vi "Test Warning to Error Handler.vi"() -> ()   [LabVIEW 2013]
uses:
  source/State Machine Support API/Select State(s)_err.vi
  source/State Machine Support API/Select State(s)_bool.vi
  <userlib>/_OpenG.lib/numeric/numeric.llb/Random Number Within Range - I32__ogtk.vi
panel:
  in  "Include Call Chain":bool
  in  "Generate Error":bool
  in  "Generate Warning":bool
  out "Previous Arguments":string
  out "Previous States":string
  out "Error message":string
  in  "Exit":bool
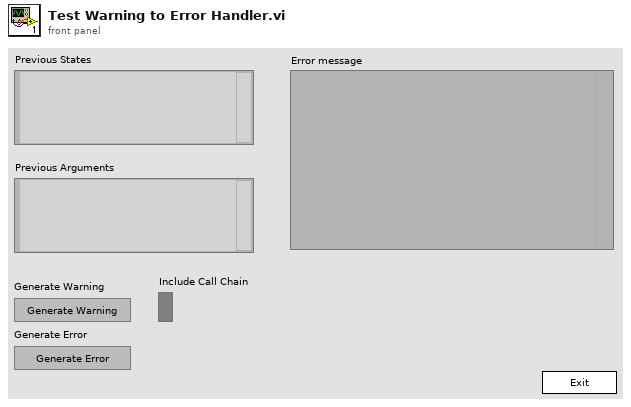
[diagram p1: front panel]
types:
  T1 = enum32{"Invalid", "Standard", "Closed", "Hidden", "Minimized", "Maximized"}
  T2 = enum32{"invalid app kind", "Development System", "Run Time System", "Student Edition", "Embedded LabVIEW", "Evaluation", "Custom"}
  T3 = cluster{"Core":cluster{"Current VI Reference":refnum<vi>, "Close Panel on Exit?":bool}, "Your Boolean data":bool, "Your string data":string}
  T4 = cluster{"Current VI Reference":refnum<vi>, "Close Panel on Exit?":bool}
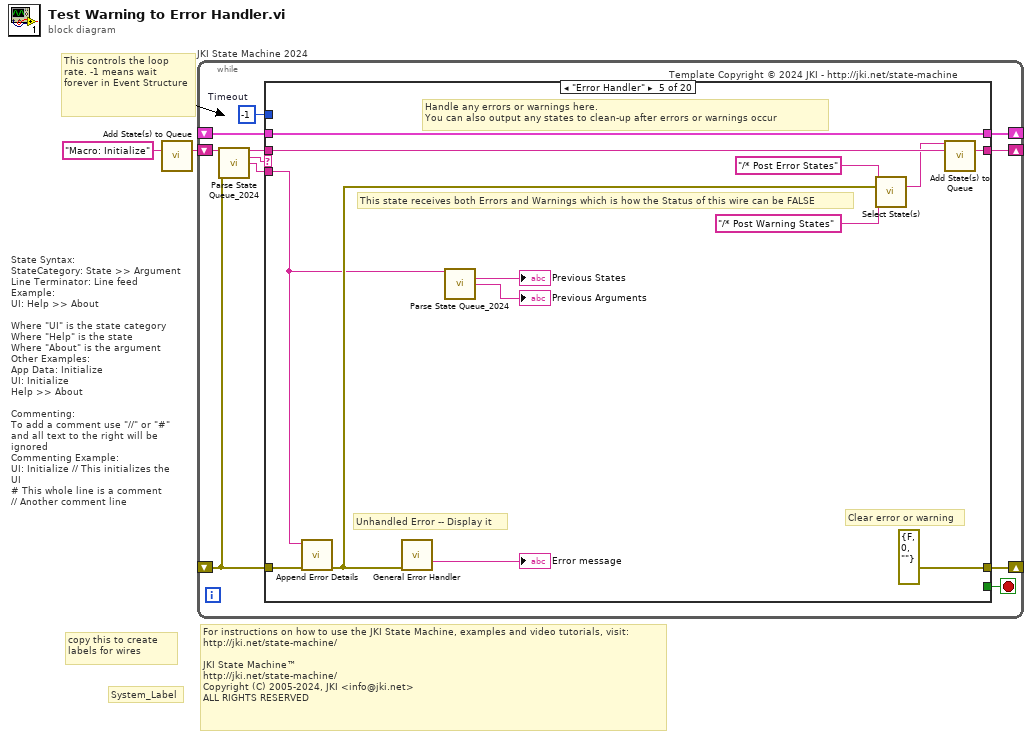
[diagram p0: block diagram]
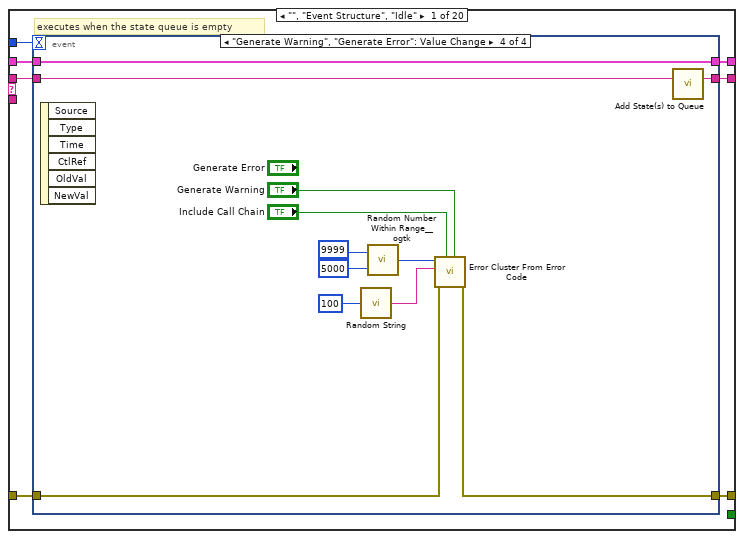
[diagram p2: hidden frame]
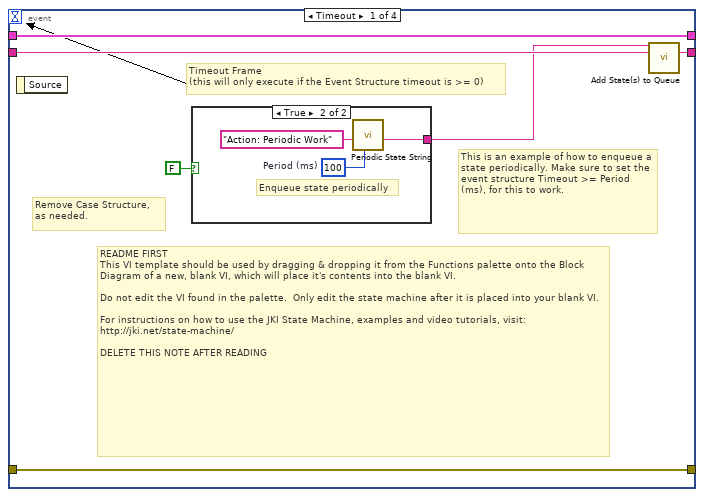
[diagram p3: hidden frame]
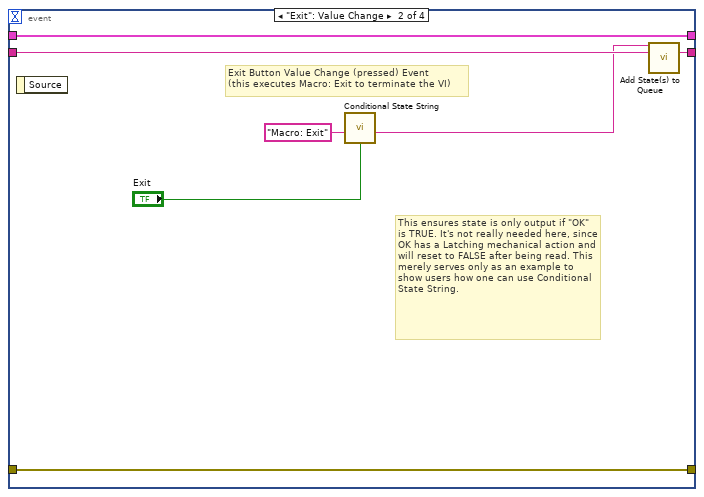
[diagram p5: hidden frame]
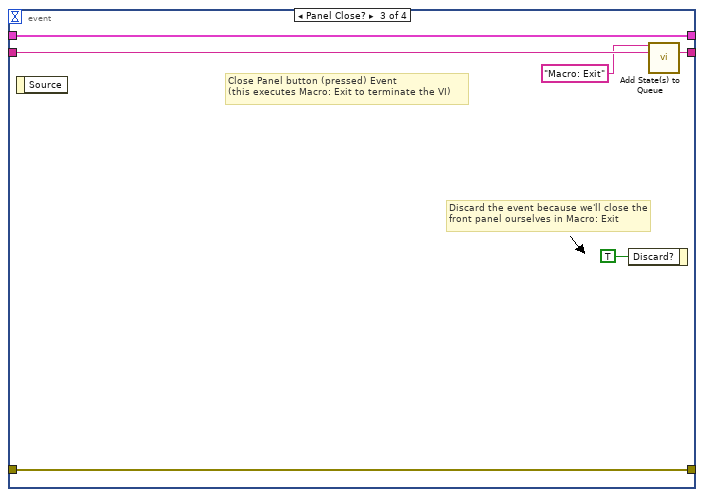
[diagram p6: hidden frame]
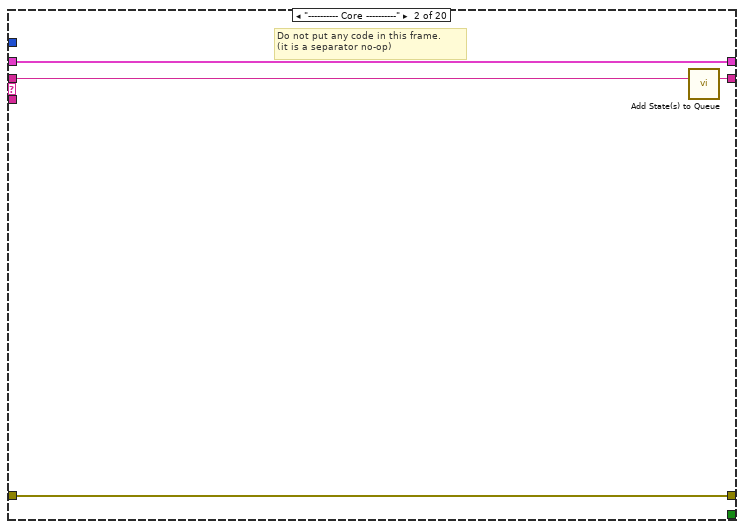
[diagram p7: hidden frame]
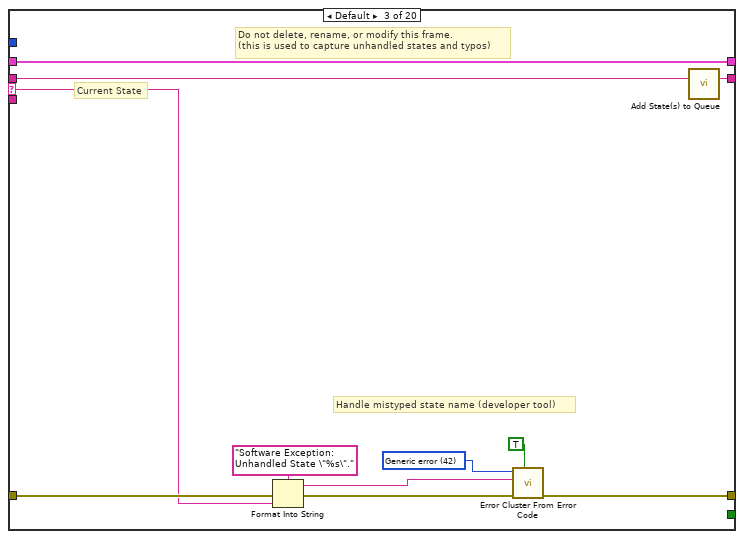
[diagram p8: hidden frame]
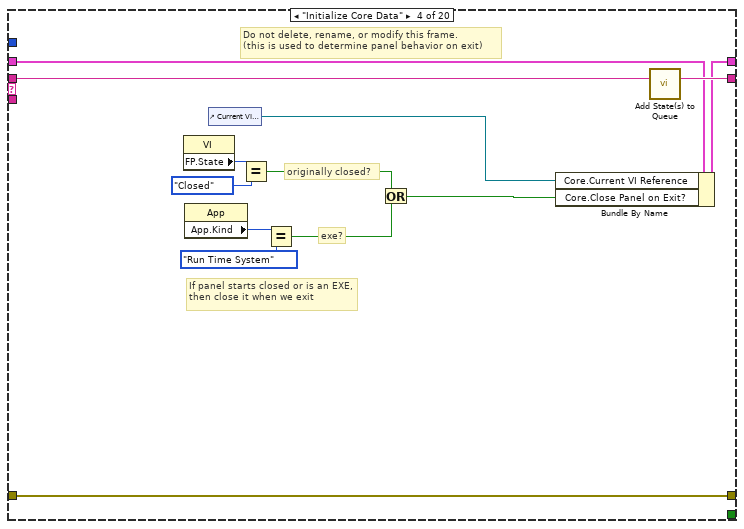
[diagram p9: hidden frame]
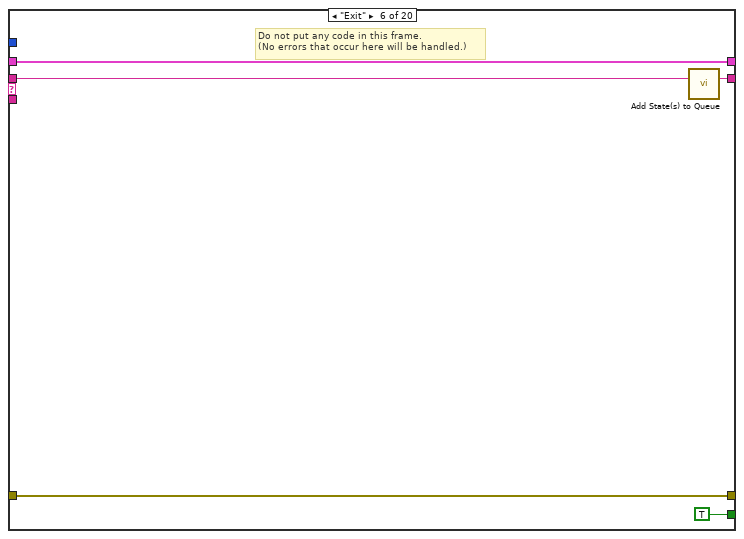
[diagram p10: hidden frame]
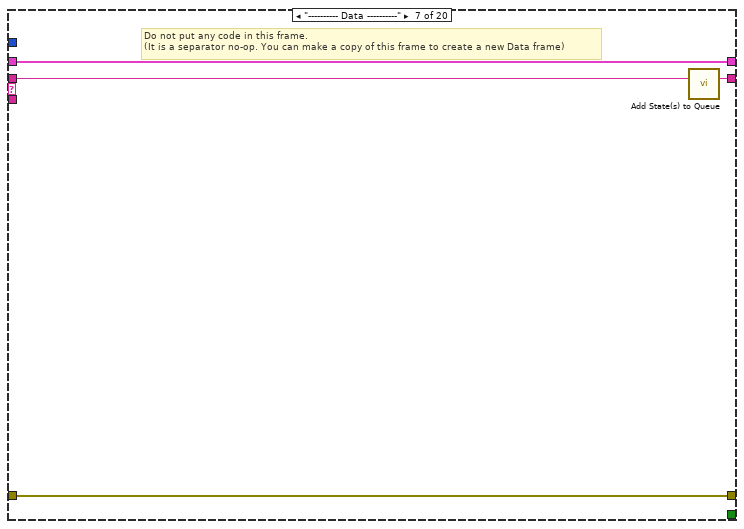
[diagram p11: hidden frame]
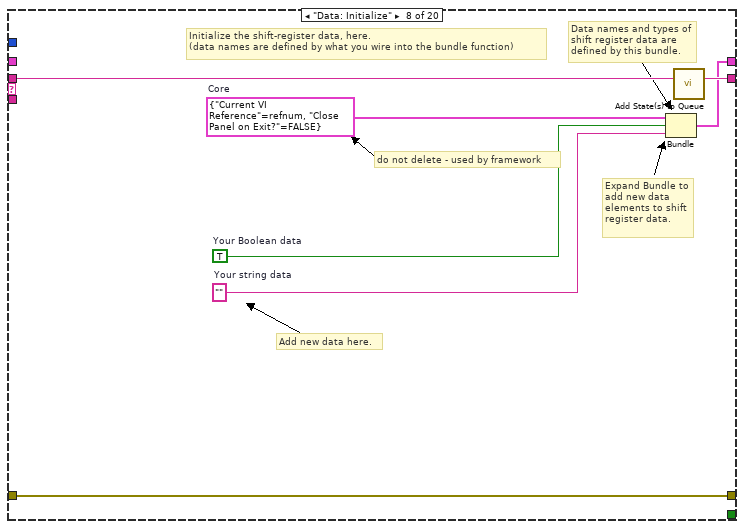
[diagram p12: hidden frame]
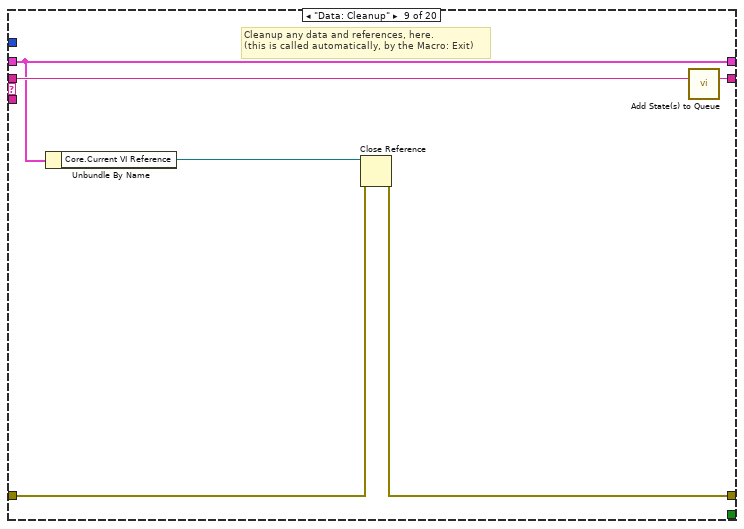
[diagram p13: hidden frame]
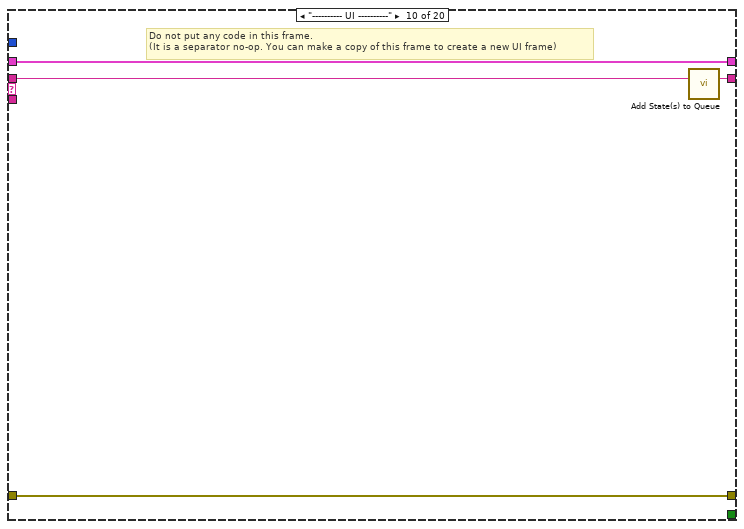
[diagram p14: hidden frame]
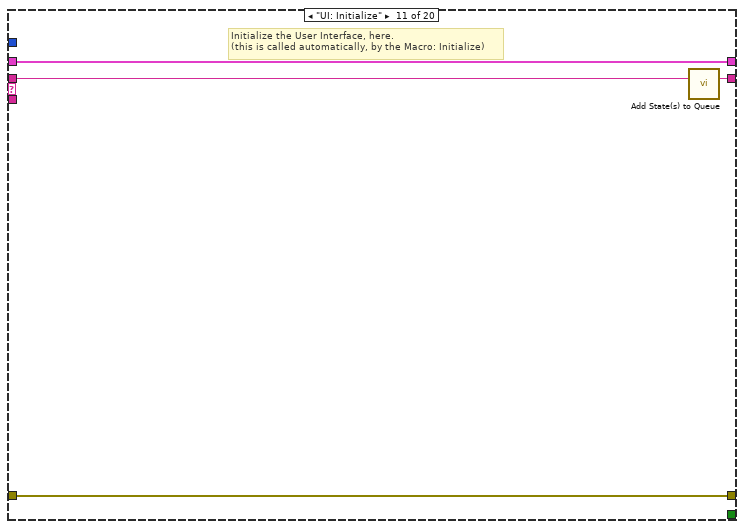
[diagram p15: hidden frame]
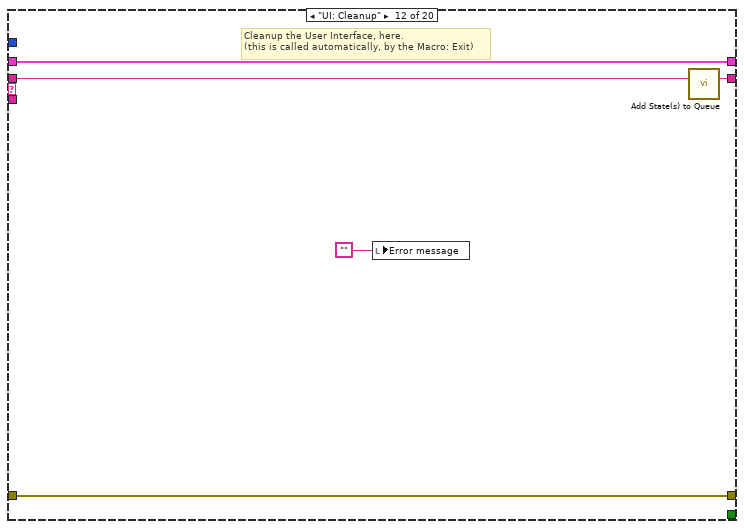
[diagram p16: hidden frame]
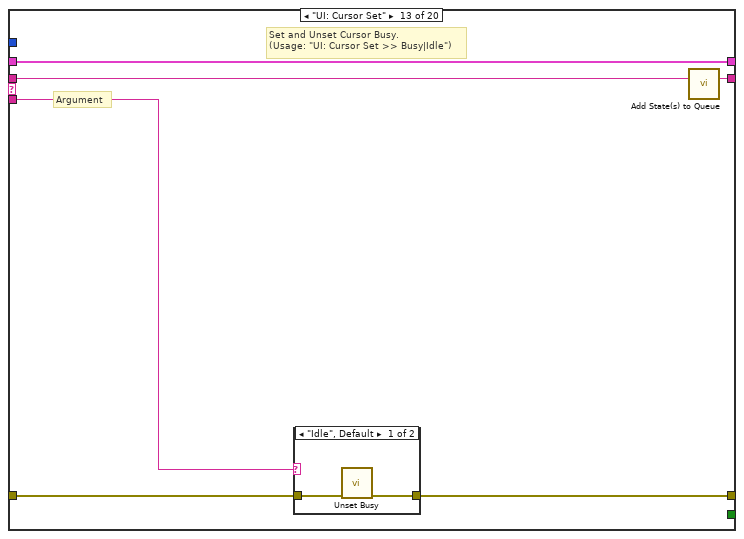
[diagram p17: hidden frame]
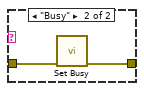
[diagram p18: hidden frame]
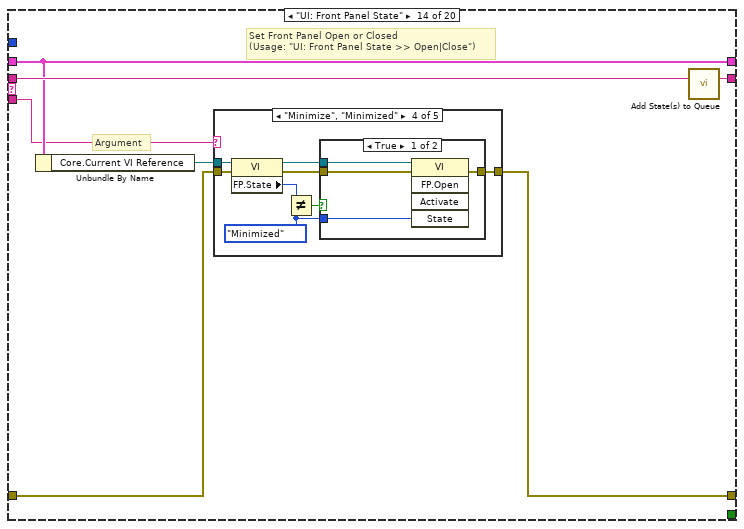
[diagram p19: hidden frame]
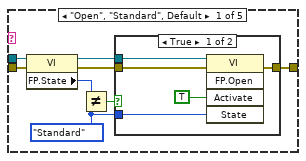
[diagram p20: hidden frame]
diagram:
  # "For instructions on how to use the JKI State Machine, examples and video tutorials, visit:\nhttp://jki.net/state-machine/\n\nJKI State Machine™\nhttp://jki.net/state-machine/\nCopyright (C) 2005-2024, JKI <info@jki.net>\nALL RIGHTS RESERVED"
  # "State Syntax:\nStateCategory: State >> Argument\nLine Terminator: Line feed\nExample:\nUI: Help >> About\n\nWhere \"UI\" is the state category\nWhere \"Help\" is the state\nWhere \"About\" is the argument\nOther Examples:\nApp Data: Initialize\nUI: Initialize\nHelp >> About\n\nCommenting:\nTo add a comment use \"//\" or \"#\" and all text to the right will be ignored\nCommenting Example:\nUI: Initialize // This initializes the UI\n# This whole line is a comment\n// Another comment line"
  # "copy this to create labels for wires"
  # "This controls the loop rate. -1 means wait forever in Event Structure"
  # "System_Label"
  n1 = call "Add State(s) to Queue.vi"("State(s) in (\"\")"="Macro: Initialize") -> ("States Out"=w1:string)  [unwired: 14 in]
  n2 = while "JKI State Machine 2024" {
    shift-right: [w6] -> _
    shift-left: _ -> [w5]
    shift-right: [w9] -> _
    shift-left: _ -> [w3]
    shift-right: [w8] -> _
    shift-left: w1 -> [w10]
    stop <- w7 stop-if-true
    w4 = -1  # Timeout
    # "Template Copyright © 2024 JKI - http://jki.net/state-machine"
    n3 = call "Parse State Queue_2024.vi"("State Queue"=w10, "Error In (no error)"=w3) -> ("Remaining States"=w12:string, "Current State"=w13:string, "Arguments"=w11:string)  [unwired: 11 in]
    n4 = case shown="\"Error Handler\"" w13 {
      selector: w13 -> [_ _ w59 _ _ _ _ _ _ _ _ _ _ _ _ _ _ _ _ _]
      tunnel: w12 -> [w20 w58 w63 w82 w95 w100 w104 w111 w117 w121 w125 w130 w136 w147 w216 w221 w230 w234 w238 w242]
      tunnel: w11 -> [_ _ _ _ w85 _ _ _ _ _ _ _ w131 w141 _ _ _ _ _ _]
      tunnel: w5 -> [w18 w55 w61 w75 w92 w98 w101 _ w112 w118 w123 w128 w134 w143 w213 w218 w228 w231 w235 w239]
      tunnel: [w17 w56 w65 w79 errorcluster {"status"=FALSE, "code"=0, "source"=""} ("error out") w97 w102 w108 w113 w119 w122 w127 w132 w144 w214 w219 w225 w232 w236 w240] -> w9
      tunnel: w3 -> [w14 w56 w64 w79 w91 w97 w102 w108 w114 w119 w122 w127 w133 w145 w214 w219 w225 w232 w236 w240]
      tunnel: [w19 w57 w62 w81 w94 w99 w103 w110 w116 w120 w124 w129 w135 w146 w215 w220 w229 w233 w237 w241] -> w8
      tunnel: [_ _ _ _ _ TRUE _ _ _ _ _ _ _ _ _ _ _ _ _ _] -> w7
      tunnel: [w16 w55 w61 w80 w92 w98 w101 w109 w112 w118 w123 w128 w134 w143 w213 w218 w228 w231 w235 w239] -> w6
      tunnel: w4 -> [w15 _ _ _ _ _ _ _ _ _ _ _ _ _ _ _ _ _ _ _]
      frame "", "Event Structure", "Idle" {
        # "executes when the state queue is empty"
        n5 = event shown="[3] \"Generate Warning\", \"Generate Error\": Value Change" {
          selector: _ -> [_ _ _ _]
          dyn-events: _ -> [_ _ _ _]
          timeout: w15 -> [_ _ _ _]
          tunnel: w20 -> [w26 w36 w42 w54]
          tunnel: [w25 w35 w41 w53] -> w19
          tunnel: w18 -> [w23 w33 w39 w52]
          tunnel: [w24 w34 w40 w48] -> w17
          tunnel: w14 -> [w24 w34 w40 w49]
          tunnel: [w23 w33 w39 w52] -> w16
          event Timeout {
            # "Remove Case Structure, as needed."
            # "This is an example of how to enqueue a state periodically. Make sure to set the event structure Timeout >= Period (ms), for this to work."
            # "README FIRST\nThis VI template should be used by dragging & dropping it from the Functions palette onto the Block Diagram of a new, blank VI, which will place it's contents into the blank VI.\n\nDo not edit the VI found in the palette.  Only edit the state machine after it is placed into your blank VI.\n\nFor instructions on how to use the JKI State Machine, examples and video tutorials, visit:\nhttp://jki.net/state-machine/\n\nDELETE THIS NOTE AFTER READING"
            # "Timeout Frame\n(this will only execute if the Event Structure timeout is >= 0)"
            n6 = event-data() -> ()  [unwired: 1 in, 1 out]
            n7 = case shown="True" FALSE {
              tunnel: [_ w29] -> w22
              frame False {
              }
              frame True {
                w27 = u32 100  # Period (ms)
                # "Enqueue state periodically"
                n8 = call "Periodic State String.vi"("Period (ms)"=w27, "State"="Action: Periodic Work") -> ("State Out"=w29:string)  [unwired: 9 in]
              }
            }
            n9 = call "Add State(s) to Queue.vi"("State(s) in Front (\"\")"=w22, "State(s) in (\"\")"=w26) -> ("States Out"=w25:string)  [unwired: 13 in]
          }
          event "Exit": Value Change {
            # "This ensures state is only output if \"OK\" is TRUE. It's not really needed here, since OK has a Latching mechanical action and will reset to FALSE after being read. This merely serves only as an example to show users how one can use Conditional State String."
            # "Exit Button Value Change (pressed) Event\n(this executes Macro: Exit to terminate the VI)"
            n10 = event-data() -> ()  [unwired: 1 in, 1 out]
            n11 = call "Conditional State String.vi"("Do State(s)?"="Exit", "State"="Macro: Exit") -> ("State Out"=w30:string)  [unwired: 7 in]
            n12 = call "Add State(s) to Queue.vi"("State(s) in Front (\"\")"=w30, "State(s) in (\"\")"=w36) -> ("States Out"=w35:string)  [unwired: 13 in]
          }
          event Panel Close? {
            # "Discard the event because we'll close the front panel ourselves in Macro: Exit"
            # "Close Panel button (pressed) Event\n(this executes Macro: Exit to terminate the VI)"
            n13 = event-data() -> ()  [unwired: 1 in, 1 out]
            n14 = event-data("Discard?"=TRUE) -> ()  [unwired: 1 in, 1 out]
            n15 = call "Add State(s) to Queue.vi"("State(s) in Front (\"\")"="Macro: Exit", "State(s) in (\"\")"=w42) -> ("States Out"=w41:string)  [unwired: 13 in]
          }
          event "Generate Warning", "Generate Error": Value Change {
            n16 = event-data() -> ()  [unwired: 1 in, 6 out]
            n17 = call "Random String.vi"("Length"=100) -> ("ASCII"=w44:string)  [unwired: 4 in]
            n18 = call-poly <userlib>:"Random Number Within Range__ogtk.vi"("High"=9999, "Low"=5000) -> ("Random Number"=w45:i32)  [unwired: 3 in]
            n19 = call <vilib>:"Error Cluster From Error Code.vi"("is warning? (False)"="Generate Warning", "show call chain? (False)"="Include Call Chain", "error in (no error)"=w49, "error message (\"\")"=w44, "error code (0)"=w45) -> ("error out"=w48:errorcluster)  [unwired: 4 in]
            n20 = call "Add State(s) to Queue.vi"("State(s) in (\"\")"=w54) -> ("States Out"=w53:string)  [unwired: 14 in]
          }
        }
      }
      frame "---------- Core ----------" {
        # "Do not put any code in this frame.\n(it is a separator no-op)"
        n21 = call "Add State(s) to Queue.vi"("State(s) in (\"\")"=w58) -> ("States Out"=w57:string)  [unwired: 14 in]
      }
      frame Default {
        w68 = 42 items=["No error", "Argument error", "Memory is full", "Out of zone", "End of file", "File already open", "Generic file I/O error", "File not found", "File permission error", "Disk is full", "Duplicate path", "Too many files open", "System feature not enabled", "Resource file not found", "Cannot add resource", "Resource not found", "Image not found", "Image memory error", "Pen does not exist", "Config type invalid", "Config token not found", "Config parse error", "Config memory error", "Bad external code format", "Bad external code offset", "External code not present", "Null window", "Destroy window error", "Null menu", "Print aborted", "Bad print record", "Print driver error", "Windows error during printing", "Memory error during printing", "Print dialog error", "Generic print error", "Invalid device refnum", "Device not found", "Device parameter error", "Device unit error", "Cannot open device", "Device call aborted", "Generic error", "Cancelled by user", "Object ID too low", "Object ID too high", "Object not in heap", "Unknown heap", "Unknown object (invalid DefProc)", "Unknown object (DefProc not in table)", "Message out of range", "Invalid (null) method", "Unknown message", "Manager call not supported", "Bad address", "Network operation in progress", "Network operation timed out", "Connection is busy", "Network attribute not supported", "Network error", "Address in use", "System out of memory", "Connection aborted", "Connection refused", "Not connected", "Already connected", "Connection closed", "Initialization error (interapplication manager)", "Bad occurrence", "Wait on unbound occurrence handler", "Occurrence queue overflow", "Datalog type conflict", "Unused", "Unrecognized type (interapplication manager)", "Memory corrupt", "Failed to make temporary DLL", "Old CIN version", "Drag socket not found", "Failed to load drop-object", "Failed to register OLE object", "Failed to release OLE object", "Format specifier type mismatch", "Unknown format specifier", "Too few format specifiers", "Too many format specifiers", "Scan failed", "Newer CIN version", "Error converting to variant", "Runtime menu error", "Password tampered", "Variant attribute not found", "Incompatible variant data type", "Event data is not available", "Event Store is not present", "Occurrence is not found", "Event Queue is not created", "Event info is not available", "Refnum passed is NULL", "Error retrieving Class GUID", "Error retrieving CoClass GUID", "Error retrieving TypeLib GUID.", "Bad built application magic bytes.", "Specific driver is different from the specific driver associated with the Logical Name.", "There is no session opened to the class driver.", "Max Error", "MAX - Error with config objects", "MAX - Error loading configuration", "MAX - Group not supported"]
        # "Current State"
        # "Do not delete, rename, or modify this frame.\n(this is used to capture unhandled states and typos)"
        # "Handle mistyped state name (developer tool)"
        n22 = Format Into String(format string="Software Exception: Unhandled State \"%s\"." ("message"), error in=w64, w59) -> (resulting string=w67:string, error out=w66:errorcluster)  [unwired: 1 in]
        n23 = call <vilib>:"Error Cluster From Error Code.vi"("show call chain? (False)"=TRUE, "error in (no error)"=w66, "error message (\"\")"=w67, "error code (0)"=w68) -> ("error out"=w65:errorcluster)  [unwired: 5 in]
        n24 = call "Add State(s) to Queue.vi"("State(s) in (\"\")"=w63) -> ("States Out"=w62:string)  [unwired: 14 in]
      }
      frame "Initialize Core Data" {
        # "Do not delete, rename, or modify this frame.\n(this is used to determine panel behavior on exit)"
        # "originally closed?"
        # "exe?"
        # "If panel starts closed or is an EXE, then close it when we exit"
        n25 = property class="VI"() -> ("FP.State"=w72:T1)  [unwired: 2 in, 2 out]
        n26 = property class="App"() -> ("App.Kind"=w78:T2)  [unwired: 2 in, 2 out]
        n27 = control-ref of="Current VI Reference"() -> (w73:refnum<vi>)
        n28 = Equal?(x=w72, y=T1."Closed" ("Front Panel Window:State")) -> (x = y?=w70:bool)
        n29 = Equal?(x=w78, y=T2."Run Time System" ("Application:Kind")) -> (x = y?=w76:bool)
        n30 = Or(x=w70, y=w76) -> (x .or. y?=w74:bool)
        n31 = Bundle By Name(cluster=w75, "Core.Current VI Reference"=w73, "Core.Close Panel on Exit?"=w74) -> (w80:T3)
        n32 = call "Add State(s) to Queue.vi"("State(s) in (\"\")"=w82) -> ("States Out"=w81:string)  [unwired: 14 in]
      }
      frame "Error Handler" {
        # "This state receives both Errors and Warnings which is how the Status of this wire can be FALSE"
        # "Unhandled Error -- Display it"
        # "Handle any errors or warnings here.\nYou can also output any states to clean-up after errors or warnings occur"
        # "Clear error or warning"
        n33 = call "Append Error Details.vi"("error in (no error)"=w91, "Previous State and Argument(s)"=w85) -> ("error out"=w90:errorcluster)  [unwired: 9 in]
        n34 = call <vilib>:"General Error Handler.vi"("error in (no error)"=w90) -> ("message"=→"Error message":string)  [unwired: 10 in, 4 out]
        n35 = call "Parse State Queue_2024.vi"("State Queue"=w85) -> ("Current State"=→"Previous States":string, "Arguments"=→"Previous Arguments":string)  [unwired: 12 in, 1 out]
        n36 = call-poly "Select State(s).vi"("State(s) if True (\"\")"="/* Post Error States", "Select"=w90, "State(s) if False (\"\")"="/* Post Warning States") -> ("States Out"=w88:string)  [unwired: 12 in]
        n37 = call "Add State(s) to Queue.vi"("State(s) in Front (\"\")"=w88, "State(s) in (\"\")"=w95) -> ("States Out"=w94:string)  [unwired: 13 in]
      }
      frame "Exit" {
        # "Do not put any code in this frame.\n(No errors that occur here will be handled.)"
        n38 = call "Add State(s) to Queue.vi"("State(s) in (\"\")"=w100) -> ("States Out"=w99:string)  [unwired: 14 in]
      }
      frame "---------- Data ----------" {
        # "Do not put any code in this frame.\n(It is a separator no-op. You can make a copy of this frame to create a new Data frame)"
        n39 = call "Add State(s) to Queue.vi"("State(s) in (\"\")"=w104) -> ("States Out"=w103:string)  [unwired: 14 in]
      }
      frame "Data: Initialize" {
        w105 = T4 {"Current VI Reference"=refnum, "Close Panel on Exit?"=FALSE}  # Core
        w107 = TRUE  # Your Boolean data
        w106 = ""  # Your string data
        # "do not delete - used by framework"
        # "Expand Bundle to add new data elements to shift register data."
        # "Add new data here."
        # "Data names and types of shift register data are defined by this bundle."
        # "Initialize the shift-register data, here.\n(data names are defined by what you wire into the bundle function)"
        n40 = Bundle("Core"=w105, "Your Boolean data"=w107, "Your string data"=w106) -> (w109:T3)  [unwired: 1 in]
        n41 = call "Add State(s) to Queue.vi"("State(s) in (\"\")"=w111) -> ("States Out"=w110:string)  [unwired: 14 in]
      }
      frame "Data: Cleanup" {
        # "Cleanup any data and references, here.\n(this is called automatically, by the Macro: Exit)"
        n42 = Unbundle By Name(w112) -> ("Core.Current VI Reference"=w115:refnum<vi>)
        n43 = Close Reference(reference=w115, error in (no error)=w114) -> (error out=w113:errorcluster)
        n44 = call "Add State(s) to Queue.vi"("State(s) in (\"\")"=w117) -> ("States Out"=w116:string)  [unwired: 14 in]
      }
      frame "---------- UI ----------" {
        # "Do not put any code in this frame.\n(It is a separator no-op. You can make a copy of this frame to create a new UI frame)"
        n45 = call "Add State(s) to Queue.vi"("State(s) in (\"\")"=w121) -> ("States Out"=w120:string)  [unwired: 14 in]
      }
      frame "UI: Initialize" {
        # "Initialize the User Interface, here.\n(this is called automatically, by the Macro: Initialize)"
        n46 = call "Add State(s) to Queue.vi"("State(s) in (\"\")"=w125) -> ("States Out"=w124:string)  [unwired: 14 in]
      }
      frame "UI: Cleanup" {
        # "Cleanup the User Interface, here.\n(this is called automatically, by the Macro: Exit)"
        n47 = local write "Error message"("") -> ()
        n48 = call "Add State(s) to Queue.vi"("State(s) in (\"\")"=w130) -> ("States Out"=w129:string)  [unwired: 14 in]
      }
      frame "UI: Cursor Set" {
        # "Argument"
        # "Set and Unset Cursor Busy.\n(Usage: \"UI: Cursor Set >> Busy|Idle\")"
        n49 = case shown="\"Idle\", Default" w131 {
          tunnel: w133 -> [w138 w140]
          tunnel: [w137 w139] -> w132
          frame "Idle", Default {
            n50 = call <vilib>:"Unset Busy.vi"("error in (no error)"=w138) -> ("error out"=w137:errorcluster)  [unwired: 10 in]
          }
          frame "Busy" {
            n51 = call <vilib>:"Set Busy.vi"("error in (no error)"=w140) -> ("error out"=w139:errorcluster)  [unwired: 9 in, 1 out]
          }
        }
        n52 = call "Add State(s) to Queue.vi"("State(s) in (\"\")"=w136) -> ("States Out"=w135:string)  [unwired: 14 in]
      }
      frame "UI: Front Panel State" {
        # "Argument"
        # "Set Front Panel Open or Closed\n(Usage: \"UI: Front Panel State >> Open|Close\")"
        n53 = Unbundle By Name(w143) -> ("Core.Current VI Reference"=w142:refnum<vi>)
        n54 = case shown="\"Minimize\", \"Minimized\"" w141 {
          tunnel: w145 -> [w153 w168 w179 w192 w205]
          tunnel: [w155 w169 w181 w194 w207] -> w144
          tunnel: w142 -> [w154 w166 w180 w193 w206]
          frame "Open", "Standard", Default {
            w148 = T1."Standard" ("State")
            n55 = property class="VI"(reference=w154, error in=w153) -> (reference out=w151:refnum<vi>, error out=w152:errorcluster, "FP.State"=w150:T1)
            n56 = Not Equal?(x=w150, y=w148) -> (x != y?=w149:bool)
            n57 = case shown="True" w149 {
              tunnel: [w159 w161] -> w155
              tunnel: w152 -> [w158 w161]
              tunnel: w151 -> [w157 _]
              tunnel: w148 -> [w156 _]
              frame True {
                n58 = invoke class="VI" method="FP.Open"(reference=w157, error in=w158, "Activate"=TRUE, "State"=w156) -> (error out=w159:errorcluster)  [unwired: 1 in, 4 out]
              }
              frame False {
              }
            }
          }
          frame "Close", "Closed" {
            n59 = property class="VI"(reference=w166, error in=w168) -> (reference out=w165:refnum<vi>, error out=w167:errorcluster, "FP.State"=w163:T1)
            n60 = Not Equal?(x=w163, y=T1."Closed" ("Front Panel Window:State")) -> (x != y?=w162:bool)
            n61 = case shown="True" w162 {
              tunnel: [w170 w173] -> w169
              tunnel: w167 -> [w170 w172]
              tunnel: w165 -> [_ w171]
              frame False {
              }
              frame True {
                n62 = invoke class="VI" method="FP.Close"(reference=w171, error in=w172) -> (error out=w173:errorcluster)  [unwired: 1 in, 2 out]
              }
            }
          }
          frame "Hidden", "Hide" {
            w174 = T1."Hidden" ("State")
            n63 = property class="VI"(reference=w180, error in=w179) -> (reference out=w177:refnum<vi>, error out=w178:errorcluster, "FP.State"=w176:T1)
            n64 = Not Equal?(x=w176, y=w174) -> (x != y?=w175:bool)
            n65 = case shown="True" w175 {
              tunnel: [w185 w186] -> w181
              tunnel: w178 -> [w184 w186]
              tunnel: w177 -> [w183 _]
              tunnel: w174 -> [w182 _]
              frame True {
                n66 = invoke class="VI" method="FP.Open"(reference=w183, error in=w184, "State"=w182) -> (error out=w185:errorcluster)  [unwired: 2 in, 4 out]
              }
              frame False {
              }
            }
          }
          frame "Minimize", "Minimized" {
            w187 = T1."Minimized" ("State")
            n67 = property class="VI"(reference=w193, error in=w192) -> (reference out=w190:refnum<vi>, error out=w191:errorcluster, "FP.State"=w189:T1)
            n68 = Not Equal?(x=w189, y=w187) -> (x != y?=w188:bool)
            n69 = case shown="True" w188 {
              tunnel: [w198 w199] -> w194
              tunnel: w191 -> [w197 w199]
              tunnel: w190 -> [w196 _]
              tunnel: w187 -> [w195 _]
              frame True {
                n70 = invoke class="VI" method="FP.Open"(reference=w196, error in=w197, "State"=w195) -> (error out=w198:errorcluster)  [unwired: 2 in, 4 out]
              }
              frame False {
              }
            }
          }
          frame "Maximize", "Maximized" {
            w200 = T1."Maximized" ("State")
            n71 = property class="VI"(reference=w206, error in=w205) -> (reference out=w203:refnum<vi>, error out=w204:errorcluster, "FP.State"=w202:T1)
            n72 = Not Equal?(x=w202, y=w200) -> (x != y?=w201:bool)
            n73 = case shown="True" w201 {
              tunnel: [w211 w212] -> w207
              tunnel: w204 -> [w210 w212]
              tunnel: w203 -> [w209 _]
              tunnel: w200 -> [w208 _]
              frame True {
                n74 = invoke class="VI" method="FP.Open"(reference=w209, error in=w210, "State"=w208) -> (error out=w211:errorcluster)  [unwired: 2 in, 4 out]
              }
              frame False {
              }
            }
          }
        }
        n75 = call "Add State(s) to Queue.vi"("State(s) in (\"\")"=w147) -> ("States Out"=w146:string)  [unwired: 14 in]
      }
      frame "---------- Macro ----------" {
        # "Do not put any code in this frame.\n(It is a separator no-op. You can make a copy of this frame to create a new Macro frame)"
        n76 = call "Add State(s) to Queue.vi"("State(s) in (\"\")"=w216) -> ("States Out"=w215:string)  [unwired: 14 in]
      }
      frame "Macro: Initialize" {
        w217 = "Data: Initialize\nInitialize Core Data\nUI: Initialize\nUI: Front Panel State >> Open"  # Data: Initialize Initialize Core Data UI: Initialize UI: Front Panel State >> Open
        # "Initialization Macro\n(This is called once, when the VI starts)"
        n77 = call "Add State(s) to Queue.vi"("State(s) in Front (\"\")"=w217, "State(s) in (\"\")"=w221) -> ("States Out"=w220:string)  [unwired: 13 in]
      }
      frame "Macro: Exit" {
        # "Exit Macro\n(This is called once, when the VI exits)"
        n78 = Unbundle By Name(w228) -> ("Core.Close Panel on Exit?"=w223:bool)
        n79 = call-poly "Select State(s).vi"("State(s) if True (\"\")"="UI: Front Panel State >> Close", "Select"=w223) -> ("States Out"=w222:string)  [unwired: 13 in]
        n80 = call "Add State(s) to Queue.vi"("State(s) in (\"\")"=w222, "State(s) at Back (\"\")"="UI: Cleanup\nData: Cleanup\nExit") -> ("States Out"=w226:string)  [unwired: 13 in]
        n81 = call "Add State(s) to Queue.vi"("State(s) in Front (\"\")"=w226, "State(s) in (\"\")"=w230) -> ("States Out"=w229:string)  [unwired: 13 in]
      }
      frame "---------- New Category ----------" {
        # "Template Separator\n(You can make a copy of, or modify, this frame)"
        n82 = call "Add State(s) to Queue.vi"("State(s) in (\"\")"=w234) -> ("States Out"=w233:string)  [unwired: 14 in]
      }
      frame "New Category: 1" {
        # "Your code here.\n(You can make a copy of, or modify, this frame)"
        n83 = call "Add State(s) to Queue.vi"("State(s) in (\"\")"=w238) -> ("States Out"=w237:string)  [unwired: 14 in]
      }
      frame "New Category: 2" {
        # "Your code here.\n(You can make a copy of, or modify, this frame)"
        n84 = call "Add State(s) to Queue.vi"("State(s) in (\"\")"=w242) -> ("States Out"=w241:string)  [unwired: 14 in]
      }
    }
  }
